vi "4_11.vi"() -> ()   [LabVIEW 2020]
panel:
  out "Valid":bool
  in  "Password":string
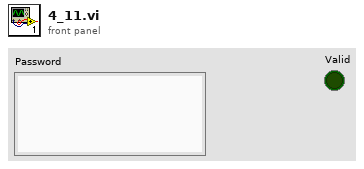
[diagram p1: front panel]
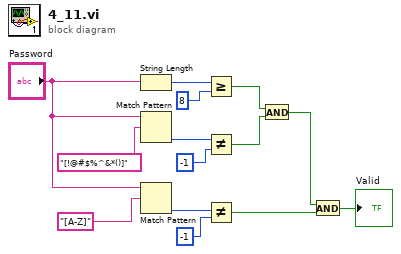
[diagram p0: block diagram]
diagram:
  n1 = String Length(string="Password") -> (length=w14:i32)
  n2 = Match Pattern(string="Password", regular expression="[!@#$%^&*()]") -> (offset past match=w11:i32)  [unwired: 1 in, 3 out]
  n3 = Match Pattern(string="Password", regular expression="[A-Z]") -> (offset past match=w6:i32)  [unwired: 1 in, 3 out]
  n4 = Greater Or Equal?(x=w14, y=8) -> (x >= y?=w5:bool)
  n5 = Not Equal?(x=w11, y=-1) -> (x != y?=w4:bool)
  n6 = Not Equal?(x=w6, y=-1) -> (x != y?=w2:bool)
  n7 = And(x=w5, y=w4) -> (x .and. y?=w3:bool)
  n8 = And(x=w3, y=w2) -> (x .and. y?=→"Valid":bool)
